vi "Lock cell.vi"(0 "Display State In":T1, 5 "Cell":cluster{"Row":i32, "Column":i32}, 7 "Lock?":bool, 9 "Container State":T6, 11 "error in (no error)":errorcluster) -> (4 "Display State Out":T1, 15 "error out":errorcluster)   [LabVIEW 2020, in "KTable.xctl"]
uses:
  KTable.xctl
  <vilib>/_xctls/Container State.ctl
  <vilib>/_xctls/XControlSupport.lvlib
  ColumnType.ctl
  ColumnSpec.ctl
  Table Properties.ctl
  Event Type.ctl
  Event Data.ctl
  Events.ctl
  State.ctl
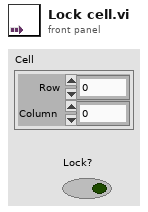
[diagram p1: front panel]
types:
  T1 = typedef "KTable.xctl/State.ctl" = cluster{"Columns":T2[], "Listbox":refnum<vi>, "Default row":string[], "Properties":T4, "Events":T5, "Locked":bool[][], "Size":cluster{"Rows":i32, "Columns":i32}, "rings":i32[][], "DefColors":u32[], "highlight row":bool}
  T2 = typedef "KTable.xctl/ColumnSpec.ctl" = cluster{"Name":string, "Type":T3, "Width":i32, "Strings":string[], "Position":enum16{"Left", "Center", "Right"}, "locked":bool, "cds":cluster{"Strings":string[]}[][], "Hide NaN":bool}
  T3 = typedef "KTable.xctl/ColumnType.ctl" = enum16{"String", "Enum", "Int", "Double", "Boolean", "Ring", "Formula", "Color"}
  T4 = typedef "KTable.xctl/Table Properties.ctl" = cluster{"Vertical scrollbar":bool, "User add/delete":bool, "Max rows":i32, "Row headers":bool}
  T5 = typedef "KTable.xctl/Events.ctl" = cluster{"Items Changed":refnum<user-event>}
  T6 = typedef "XControlSupport.lvlib/Container State.ctl" = cluster{"Indicator?":bool, "Run Mode?":bool, " Refnum":refnum<vi>}
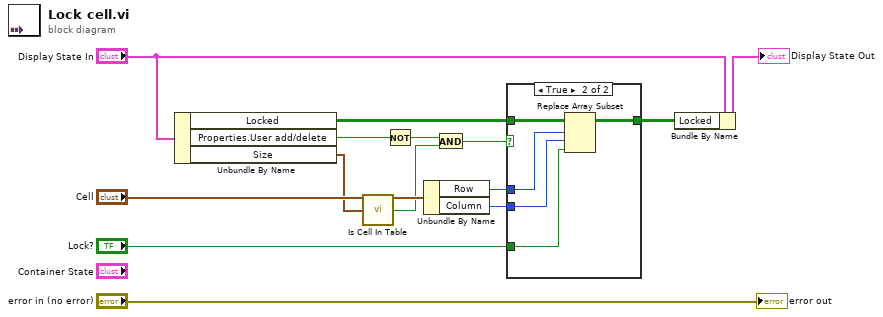
[diagram p0: block diagram]
diagram:
  n1 = Unbundle By Name("Display State In") -> ("Locked"=w13:bool[][], "Properties.User add/delete"=w4:bool, "Size"=w5:cluster{"Rows":i32, "Columns":i32})
  n2 = call "Is Cell In Table.vi"("Cell"="Cell", "Size"=w5) -> ("Cell thru"=w6:cluster{"Row":i32, "Column":i32}, "in table"=w2:bool)  [unwired: 12 in]
  n3 = Not(x=w4) -> (.not. x?=w3:bool)
  n4 = Unbundle By Name(w6) -> ("Row"=w12:i32, "Column"=w11:i32)
  n5 = And(x=w3, y=w2) -> (x .and. y?=w1:bool)
  n6 = case shown="True" w1 {
    tunnel: w13 -> [w16 w21]
    tunnel: w12 -> [_ w20]
    tunnel: w11 -> [_ w19]
    tunnel: [w16 w18] -> w9
    tunnel: "Lock?" -> [_ w17]
    frame False {
    }
    frame True {
      n7 = Replace Array Subset(array=w21, new element=w17, index (row)=w20, index (col)=w19) -> (w18:bool[][])
    }
  }
  n8 = Bundle By Name(cluster="Display State In", "Locked"=w9) -> (→"Display State Out":T1)
  "error out" <- "error in (no error)"
